vi "Setup UI.vi"(8 "error in (no error)":errorcluster, 10 "Set UI to input? (F)":bool, 11 "Translation Stage in":refnum<class "Translation Stage.lvclass">) -> (0 "error out":errorcluster, 3 "Translation Stage out":refnum<class "Translation Stage.lvclass">)   [LabVIEW 2009, in "Translation Stage.lvclass"]
doc: "Scanner::Setup is a constructor that has no parameters and faces the user. The Factory calls this VI to let the user configure this Scanner. It is dynamically dispatched in order to let the user choose the type as well as the options of the scanner."
uses:
  Translation Stage.lvclass
  Translation Stage.lvclass/Translation Stage.ctl
  Global/GPIB Numbers.vi
panel:
  in  "Specify By Sweep Rate":bool caption="Specify By Scan Time"
  in  "Coarse Only":bool
  in  "Sweep Rate":dbl[unit]=1.334e-10 min=2.1500000000000003e-12 max=2.0000000000000003e-10
  in  "Scan Time":dbl[unit]
  out "Time per Point":dbl[unit]
  in  "Discrete/Continuous":bool
  in  "Number of Path Lengths":i32=2
  in  "Calibrate Zero":bool
  in  "Send conds for first point":bool
  # "Caution: Enter the start/stop/step\nsettings above in nanoseconds!"
  # "Note:  For a continuous scan you must enter \"0\" for the dwell time above"
  # "Note:  In a continuous scan the \"Coarse Only\"\n control is forced True"
  # "PURE VIRTUAL\nMETHOD CALLED!"
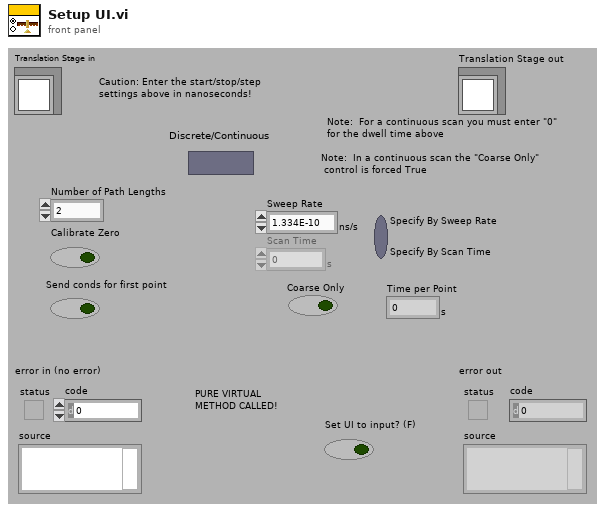
[diagram p1: front panel]
types:
  T1 = typedef "Scanner.lvclass/Range.ctl" = cluster{"xi":dbl, "xf":dbl, "dx":dbl, "Return to...?":bool, "Return to":dbl}
  T2 = typedef "GPIB Type Def.ctl" = cluster{"Name":string, "bus":dbl, "GPIB":dbl, "GPIB as string":string, "byte":i32, "VISA Resource Name":refnum<visa-resource-name>}
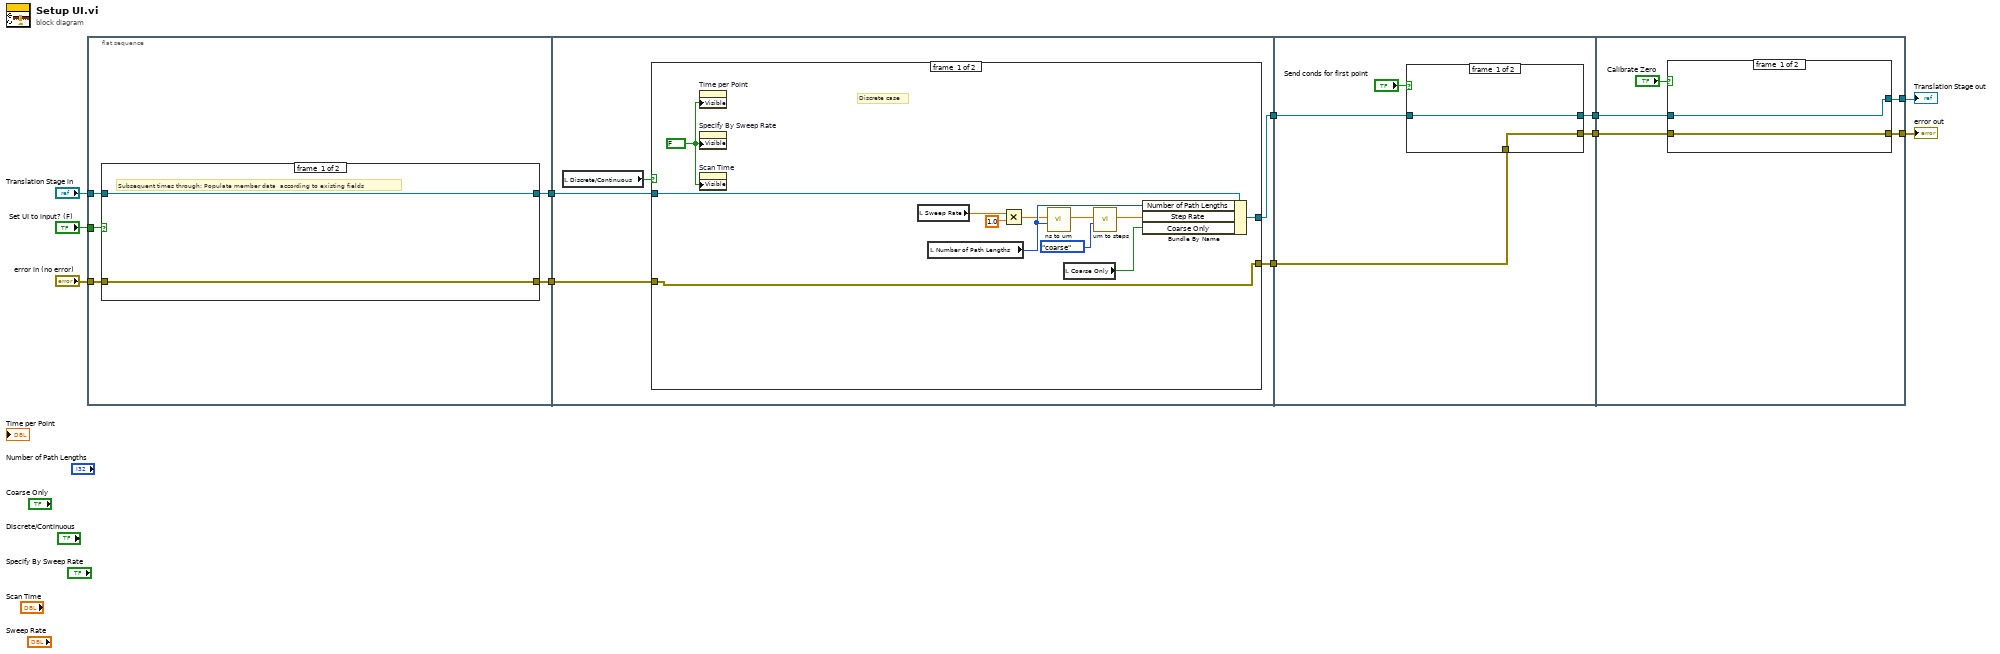
[diagram p0: block diagram]
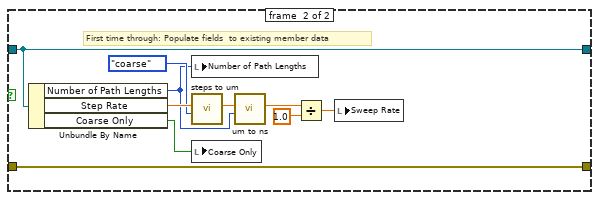
[diagram p2: hidden frame]
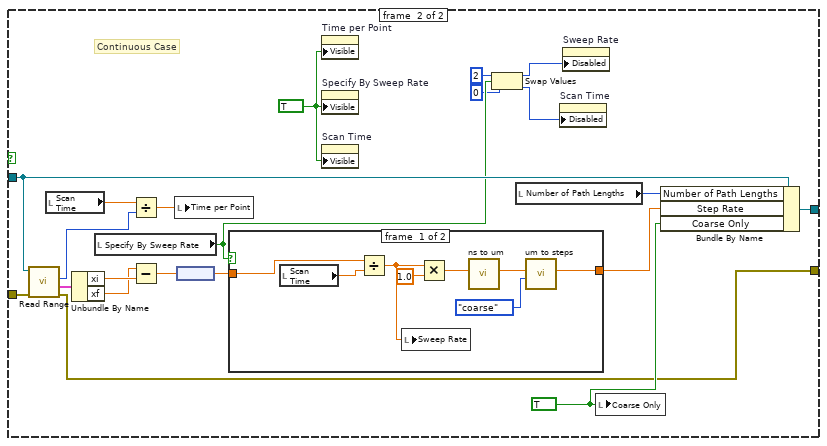
[diagram p3: hidden frame]
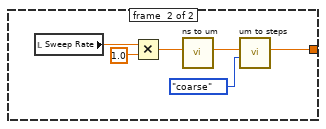
[diagram p4: hidden frame]
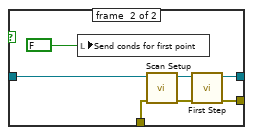
[diagram p5: hidden frame]
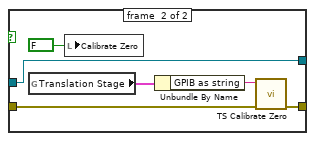
[diagram p6: hidden frame]
diagram:
  n1 = flat-sequence {
    tunnel: "Set UI to input? (F)" -> [w16]
    tunnel: "Translation Stage in" -> [w15]
    tunnel: "error in (no error)" -> [w14]
    tunnel: [w13] -> w4
    tunnel: [w12] -> w3
    tunnel: w4 -> [w32]
    tunnel: w3 -> [w31]
    tunnel: [w30] -> w2
    tunnel: [w29] -> w1
    tunnel: [w84] -> w7
    tunnel: [w83] -> w6
    tunnel: w2 -> [w82]
    tunnel: w1 -> [w81]
    tunnel: [w98] -> w5
    tunnel: [w96] -> w8
    tunnel: w7 -> [w97]
    tunnel: w6 -> [w99]
    frame #0 {
      n2 = case shown="True" w16 {
        tunnel: [w18 w28] -> w12
        tunnel: w15 -> [w18 w28]
        tunnel: [w17 w27] -> w13
        tunnel: w14 -> [w17 w27]
        frame #0 {
          # "Subsequent times through: Populate member data  according to existing fields"
        }
        frame #1 {
          # "First time through: Populate fields  to existing member data"
          n3 = Unbundle By Name(w28) -> ("Number of Path Lengths"=w22:i32, "Step Rate"=w25:dbl, "Coarse Only"=w26:bool)
          n4 = local write "Number of Path Lengths"(w22) -> ()
          n5 = call "steps to um.vi"("axis (default: fine)"=enum16{"fine", "coarse"}."coarse", "steps"=w25) -> ("position (microns)"=w23:dbl[unit])  [unwired: 7 out]
          n6 = local write "Coarse Only"(w26) -> ()
          n7 = call "um to ns.vi"("# of path lengths (def.: 2)"=w22, "position (microns)"=w23) -> ("position (ns)"=w21:dbl[unit])  [unwired: 9 out]
          n8 = Divide(x=w21, y=dbl[unit] 1.0) -> (x/y=w19:dbl)
          n9 = local write "Sweep Rate"(w19) -> ()
        }
      }
    }
    frame #1 {
      n10 = local read "Discrete/Continuous"() -> (w33:bool)
      n11 = case shown="True" w33 {
        tunnel: w32 -> [w34 w62]
        tunnel: w31 -> [w44 w57]
        tunnel: [w35 w58] -> w30
        tunnel: [w34 w52] -> w29
        frame #0 {
          w45 = FALSE
          # "Discrete case"
          n12 = property on="Time per Point" class="DigNum (strict)"("Visible"=w45) -> ()  [unwired: 2 in, 2 out]
          n13 = property on="Specify By Sweep Rate" class="Bool (strict)"("Visible"=w45) -> ()  [unwired: 2 in, 2 out]
          n14 = property on="Scan Time" class="DigNum (strict)"("Visible"=w45) -> ()  [unwired: 2 in, 2 out]
          n15 = local read "Sweep Rate"() -> (w38:dbl[unit])
          n16 = local read "Number of Path Lengths"() -> (w41:i32)
          n17 = Multiply(x=w38, y=dbl[unit] 1.0) -> (x*y=w40:dbl[unit])
          n18 = call "ns to um.vi"("number of path lengths (default: 2)"=w41, "position (ns)"=w40) -> ("position (microns)"=w42:dbl[unit])  [unwired: 9 out]
          n19 = local read "Coarse Only"() -> (w36:bool)
          n20 = call "um to steps.vi"("axis (default = fine)"=enum16{"fine", "coarse"}."coarse", "position (microns)"=w42) -> ("steps"=w37:dbl)  [unwired: 9 out]
          n21 = Bundle By Name(cluster=w44, "Number of Path Lengths"=w41, "Step Rate"=w37, "Coarse Only"=w36) -> (w35:refnum<class "Translation Stage.lvclass">)
        }
        frame #1 {
          w51 = TRUE
          w55 = TRUE
          # "Continuous Case"
          n22 = call-dynamic "Read Range.vi"("error in (no error)"=w62, "Scanner.lvclass in"=w57) -> ("error out"=w52:errorcluster, "Range"=w63:T1, "# Points"=w60:u32)  [unwired: 7 out]
          n23 = local read "Scan Time"() -> (w61:dbl[unit])
          n24 = Unbundle By Name(w63) -> ("xi"=w65:dbl, "xf"=w64:dbl)
          n25 = local read "Specify By Sweep Rate"() -> (w50:bool)
          n26 = Divide(x=w61, y=w60) -> (x/y=w59:dbl[unit])
          n27 = Subtract(x=w64, y=w65) -> (x-y=w66:dbl)
          n28 = local write "Time per Point"(w59) -> ()
          n29 = node(w66) -> (w54:dbl[unit])
          n30 = case shown="False" w50 {
            tunnel: w54 -> [w74 _]
            tunnel: [w67 w75] -> w53
            frame #0 {
              n31 = local read "Scan Time"() -> (w73:dbl[unit])
              n32 = Divide(x=w74, y=w73) -> (x/y=w68:dbl)
              n33 = local write "Sweep Rate"(w68) -> ()
              n34 = Multiply(x=w68, y=dbl[unit] 1.0) -> (x*y=w70:dbl[unit])
              n35 = call "ns to um.vi"("position (ns)"=w70) -> ("position (microns)"=w71:dbl[unit])  [unwired: 1 in, 9 out]
              n36 = call "um to steps.vi"("axis (default = fine)"=enum16{"fine", "coarse"}."coarse", "position (microns)"=w71) -> ("steps"=w67:dbl)  [unwired: 9 out]
            }
            frame #1 {
              n37 = local read "Sweep Rate"() -> (w76:dbl[unit])
              n38 = Multiply(x=w76, y=dbl[unit] 1.0) -> (x*y=w78:dbl[unit])
              n39 = call "ns to um.vi"("position (ns)"=w78) -> ("position (microns)"=w79:dbl[unit])  [unwired: 1 in, 9 out]
              n40 = call "um to steps.vi"("axis (default = fine)"=enum16{"fine", "coarse"}."coarse", "position (microns)"=w79) -> ("steps"=w75:dbl)  [unwired: 9 out]
            }
          }
          n41 = property on="Time per Point" class="DigNum (strict)"("Visible"=w51) -> ()  [unwired: 2 in, 2 out]
          n42 = property on="Specify By Sweep Rate" class="Bool (strict)"("Visible"=w51) -> ()  [unwired: 2 in, 2 out]
          n43 = property on="Scan Time" class="DigNum (strict)"("Visible"=w51) -> ()  [unwired: 2 in, 2 out]
          n44 = Swap Values(12:2 ("y"), 13:w50, 14:0 ("x")) -> (1:w47:i32, 3:w46:i32)
          n45 = local read "Number of Path Lengths"() -> (w56:i32)
          n46 = property on="Scan Time" class="DigNum (strict)"("Disabled"=w46) -> ()  [unwired: 2 in, 2 out]
          n47 = property on="Sweep Rate" class="DigNum (strict)"("Disabled"=w47) -> ()  [unwired: 2 in, 2 out]
          n48 = local write "Coarse Only"(w55) -> ()
          n49 = Bundle By Name(cluster=w57, "Number of Path Lengths"=w56, "Step Rate"=w53, "Coarse Only"=w55) -> (w58:refnum<class "Translation Stage.lvclass">)
        }
      }
    }
    frame #2 {
      n50 = case shown="True" "Send conds for first point" {
        tunnel: [w86 w91] -> w84
        tunnel: [w87 w90] -> w83
        tunnel: w82 -> [w87 w89]
        tunnel: w81 -> [w86 w88]
        frame #0 {
        }
        frame #1 {
          n51 = local write "Send conds for first point"(FALSE ("Send conds for first point to PG")) -> ()
          n52 = call-dynamic "Scan Setup.vi"("error in (no error)"=w88, "Translation Stage in"=w89) -> ("error out"=w92:errorcluster, "Translation Stage out"=w93:refnum<class "Translation Stage.lvclass">)  [unwired: 8 out]
          n53 = call-dynamic "First Step.vi"("error in (no error)"=w92, "Translation Stage.lvclass in"=w93) -> ("error out"=w91:errorcluster, "Translation Stage.lvclass out"=w90:refnum<class "Translation Stage.lvclass">)  [unwired: 8 out]
        }
      }
    }
    frame #3 {
      n54 = case shown="True" "Calibrate Zero" {
        tunnel: [w101 w102] -> w96
        tunnel: [w100 w103] -> w98
        tunnel: w99 -> [w100 w103]
        tunnel: w97 -> [w101 w104]
        frame #0 {
        }
        frame #1 {
          n55 = global read "GPIB Numbers.vi" "Translation Stage"() -> (w106:T2)
          n56 = local write "Calibrate Zero"(FALSE ("Send conds for first point to PG")) -> ()
          n57 = Unbundle By Name(w106) -> ("GPIB as string"=w105:string)
          n58 = call "TS Calibrate Zero.vi"("error out"=w104, "GPIB as string"=w105) -> ("error out 2"=w102:errorcluster)  [unwired: 9 out]
        }
      }
    }
  }
  "error out" <- w8
  "Translation Stage out" <- w5
